vi "7.5.1.vi"   [LabVIEW 2018]
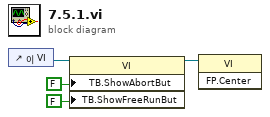
[diagram p0: block diagram]
diagram:
  n1 = control-ref of="이 VI"() -> (w4:refnum<vi>)
  n2 = property class="VI"(reference=w4, "TB.ShowAbortBut"=FALSE ("도구 모음:강제 종료 버튼 보이기"), "TB.ShowFreeRunBut"=FALSE ("도구 모음:연속 실행 버튼 보이기")) -> (reference out=w3:refnum<vi>)  [unwired: 1 in, 1 out]
  n3 = invoke class="VI" method="FP.Center"(reference=w3) -> ()  [unwired: 2 in, 3 out]
